vi "Serialport_IsRxDone.vi"(6 "应答长度检测":i32, 7 "StopFlagRef":refnum<notifier>, 8 "error in (no error)":errorcluster, 9 "应答检测":string, 10 "接收前延迟ms":u32, 11 "VISA":refnum<visa-resource-name>) -> (0 "error out":errorcluster, 1 "Rx":string, 2 "WaitTime":u32, 3 "VISA out":refnum<visa-resource-name>)   [LabVIEW 2017]
doc: "YYLL VarSystem"
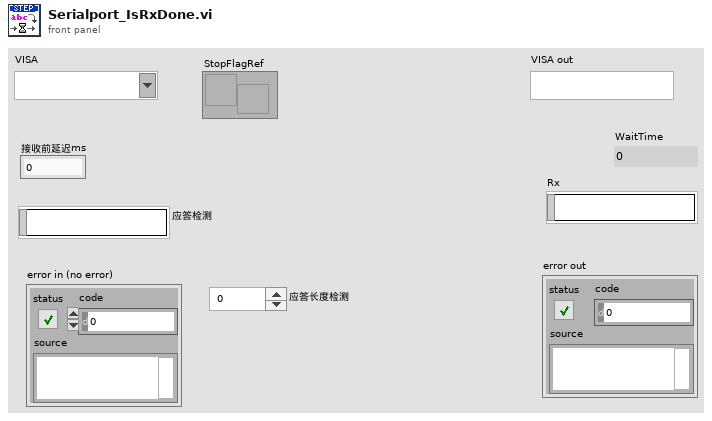
[diagram p1: front panel]
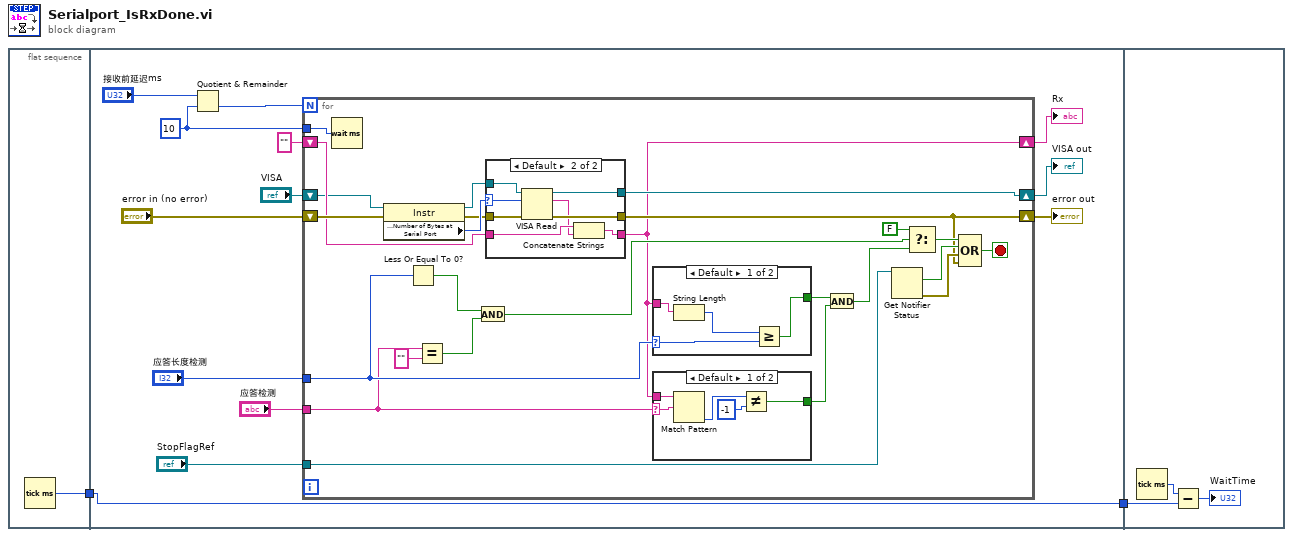
[diagram p0: block diagram]
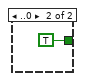
[diagram p2: hidden frame]
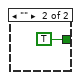
[diagram p3: hidden frame]
diagram:
  n1 = flat-sequence {
    tunnel: [w3] -> w2
    tunnel: w2 -> [w4]
    tunnel: [w4] -> w1
    tunnel: w1 -> [w65]
    frame #0 {
      n2 = Tick Count (ms)() -> (millisecond timer value=w3:u32)
    }
    frame #1 {
      w12 = u32 10 ("y")
      n3 = Quotient & Remainder(x="接收前延迟ms", y=w12) -> (floor(x/y)=w11:u32)  [unwired: 1 out]
      n4 = for {
        N: w11 -> [_]
        tunnel: "StopFlagRef" -> [w41]
        shift-right: [w35] -> w15
        shift-left: "VISA" -> [w33]
        tunnel: w12 -> [w40]
        shift-right: [w18] -> w9
        shift-left: "error in (no error)" -> [w39]
        shift-right: [w17] -> w7
        shift-left: "" -> [w34]
        tunnel: "应答检测" -> [w28]
        tunnel: "应答长度检测" -> [w29]
        stop <- w30 stop-if-true
        n5 = Wait (ms)(milliseconds to wait=w40) -> ()  [unwired: 1 out]
        n6 = property class="Instr"(reference=w33, error in=w39) -> (reference out=w36:refnum<visa-resource-name>, error out=w37:errorcluster, "Serial Settings:Number of Bytes at Serial Port"=w38:u32)
        n7 = Less Or Equal To 0?(x=w29) -> (x <= 0?=w26:bool)
        n8 = Equal?(x=w28, y="") -> (x = y?=w25:bool)
        n9 = And(x=w26, y=w25) -> (x .and. y?=w24:bool)
        n10 = case shown="Default" w38 {
          selector: w38 -> [_ w56]
          tunnel: w37 -> [w54 w61]
          tunnel: w36 -> [w55 w63]
          tunnel: [w55 w62] -> w35
          tunnel: [w54 w60] -> w18
          tunnel: w34 -> [w53 w59]
          tunnel: [w53 w58] -> w17
          frame 0 {
          }
          frame Default {
            n11 = VISA Read(VISA resource name=w63, byte count=w56, error in (no error)=w61) -> (VISA resource name out=w62:refnum<visa-resource-name>, read buffer=w57:string, error out=w60:errorcluster)  [unwired: 1 out]
            n12 = Concatenate Strings(w59, w57) -> (w58:string)
          }
        }
        n13 = case shown="Default" w29 {
          selector: w29 -> [w43 _]
          tunnel: w17 -> [w45 _]
          tunnel: [w42 TRUE] -> w32
          frame Default {
            n14 = String Length(string=w45) -> (length=w44:i32)
            n15 = Greater Or Equal?(x=w44, y=w43) -> (x >= y?=w42:bool)
          }
          frame ..0 {
          }
        }
        n16 = case shown="Default" w28 {
          selector: w28 -> [w50 _]
          tunnel: w17 -> [w51 _]
          tunnel: [w47 TRUE] -> w31
          frame Default {
            n17 = Match Pattern(string=w51, regular expression=w50) -> (offset past match=w49:i32)  [unwired: 1 in, 3 out]
            n18 = Not Equal?(x=w49, y=-1) -> (x != y?=w47:bool)
          }
          frame "" {
          }
        }
        n19 = And(x=w32, y=w31) -> (x .and. y?=w21:bool)
        n20 = Get Notifier Status(notifier=w41) -> (current notification=w20:bool, error out=w19:errorcluster)  [unwired: 1 in, 3 out]
        n21 = Select(t=FALSE, s=w24, f=w21) -> (s? t:f=w22:bool)
        n22 = Compound Arithmetic op=OR(w22, w20, w19, w18) -> (w30:bool)
      }
      "VISA out" <- w15
      "error out" <- w9
      "Rx" <- w7
    }
    frame #2 {
      n23 = Tick Count (ms)() -> (millisecond timer value=w66:u32)
      n24 = Subtract(x=w66, y=w65) -> (x-y=→"WaitTime":u32)
    }
  }
